vi "SPI Init.vi"(8 "Error In":errorcluster, 11 "SPI Configuration In":T1={"CLK Frequency (Hz)"=250000, "CPOL"=FALSE, "CPHA"=FALSE, "CS Channel"="", "CLK Channel"="", "MOSI Channel"="", "MISO Channel"="", "Active CS"=FALSE, "Dig In Task"="", "Dig Out Task"=""} {"CLK Frequency (Hz)" format="%#.6p"}) -> (0 "Error Out":errorcluster, 3 "SPI Configuration Out":T1={"CLK Frequency (Hz)"=250000, "CPOL"=FALSE, "CPHA"=FALSE, "CS Channel"="", "CLK Channel"="", "MOSI Channel"="", "MISO Channel"="", "Active CS"=FALSE, "Dig In Task"="", "Dig Out Task"=""} {"CLK Frequency (Hz)" format="%#.6p"})   [LabVIEW 2016, in "SPIVI.lvlib"]
uses:
  SPIVI.lvlib
  Typedefs/SPI Configuration.ctl
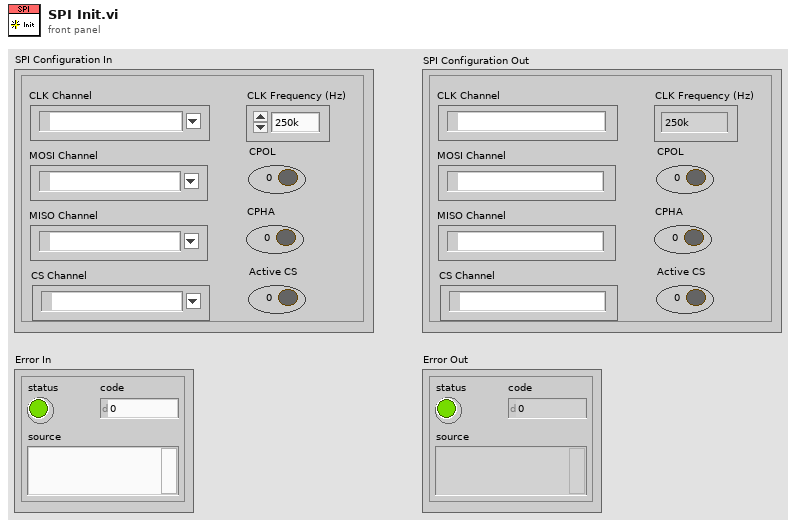
[diagram p1: front panel]
types:
  T1 = typedef "SPIVI.lvlib/SPI Configuration.ctl" = cluster{"CLK Frequency (Hz)":u32, "CPOL":bool, "CPHA":bool, "CS Channel":tag, "CLK Channel":tag, "MOSI Channel":tag, "MISO Channel":tag, "Active CS":bool, "Dig In Task":refnum<k21>, "Dig Out Task":refnum<k21>}
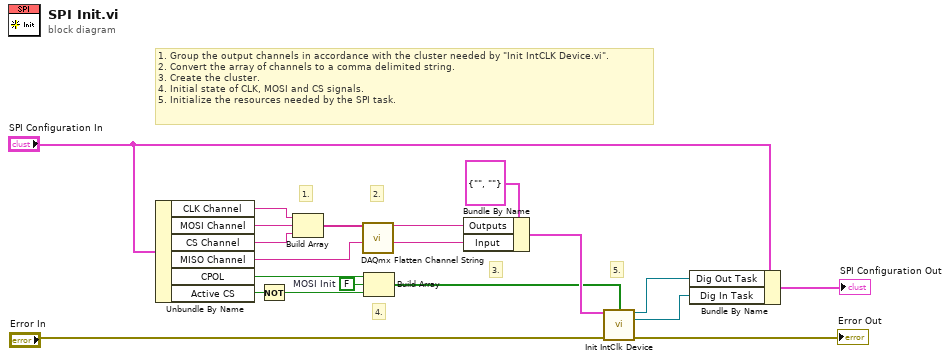
[diagram p0: block diagram]
diagram:
  w2 = FALSE  # MOSI Init
  # "5."
  # "4."
  # "3."
  # "2."
  # "1."
  # "1. Group the output channels in accordance with the cluster needed by \"Init IntCLK Device.vi\".\n2. Convert the array of channels to a comma delimited string.\n3. Create the cluster.\n4. Initial state of CLK, MOSI and CS signals.\n5. Initialize the resources needed by the SPI task."
  n1 = Unbundle By Name("SPI Configuration In") -> ("CLK Channel"=w13:tag, "MOSI Channel"=w12:tag, "CS Channel"=w11:tag, "MISO Channel"=w10:tag, "CPOL"=w9:bool, "Active CS"=w1:bool)
  n2 = Not(x=w1) -> (.not. x?=w15:bool)
  n3 = Build Array(w13, w12, w11) -> (w18:tag[])
  n4 = call <vilib>:"DAQmx Flatten Channel String.vi"("names in"=w18) -> ("names out"=w17:string)  [unwired: 13 in, 1 out]
  n5 = Build Array(w9, w2, w15) -> (w14:bool[])
  n6 = Bundle By Name(cluster=cluster{"Outputs":tag, "Input":tag} {"Outputs"="", "Input"=""} ("Physical Channels"), "Outputs"=w17, "Input"=w10) -> (w16:cluster{"Outputs":tag, "Input":tag})
  n7 = call "Init IntClk Device.vi"("Physical Channels"=w16, "error in (no error)"="Error In", "Initial output states"=w14) -> ("Dig out task out"=w4:refnum<k21>, "Dig in task out"=w3:refnum<k21>, "error out"=→"Error Out":errorcluster)  [unwired: 10 in]
  n8 = Bundle By Name(cluster="SPI Configuration In", "Dig Out Task"=w4, "Dig In Task"=w3) -> (→"SPI Configuration Out":T1)
